vi "Main.vi"() -> ()   [LabVIEW 2010]
uses:
  vi.lib/Front Panel Layout/NI_SE_Front Panel Layout.lvlib
panel:
  in  "c":bool
  in  "b":bool
  in  "a":bool
  in  "Power":bool
  out "Sensor Data":dbl[](graph)
  in  "Config Keyword":string="small1"
  in  "cancel":bool
  in  "ok":bool
  # "The following values can be used for Config Keyword:\nsmall1\nsmall2\nlarge1"
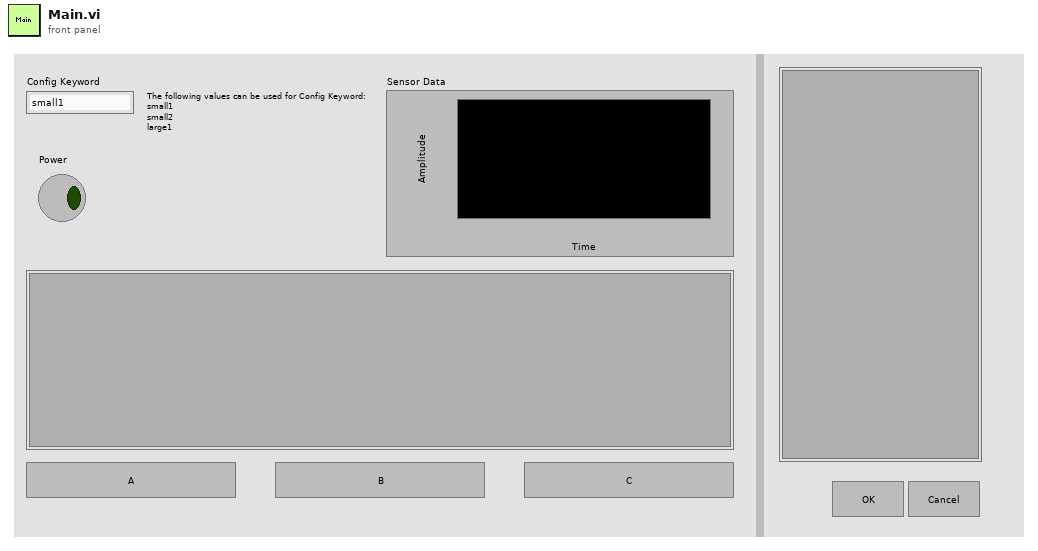
[diagram p1: front panel]
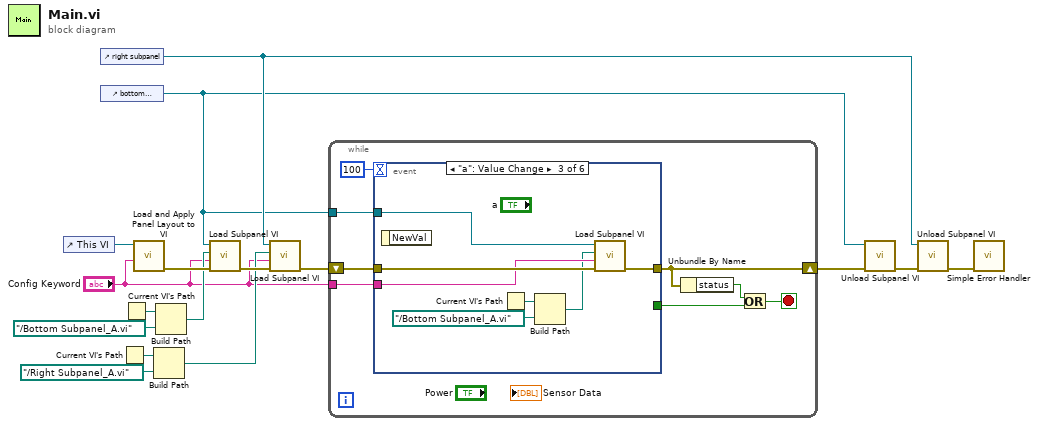
[diagram p0: block diagram]
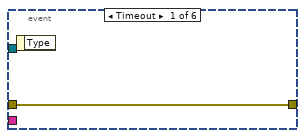
[diagram p2: hidden frame]
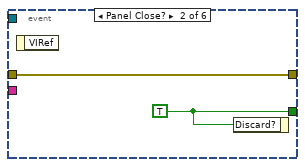
[diagram p3: hidden frame]
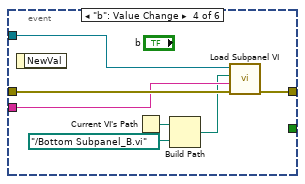
[diagram p4: hidden frame]
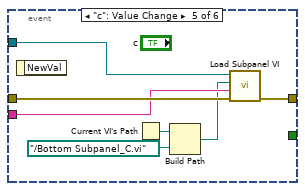
[diagram p5: hidden frame]
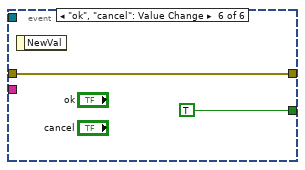
[diagram p6: hidden frame]
diagram:
  n1 = control-ref of="This VI"() -> (w16:refnum<vi>)
  n2 = control-ref of="right subpanel"() -> (w4:refnum<vi>)
  n3 = control-ref of="bottom subpanel"() -> (w3:refnum<vi>)
  n4 = Current VI's Path() -> (path=w7:path)
  n5 = Current VI's Path() -> (path=w15:path)
  n6 = call "Load and Apply Panel Layout to VI.vi"("keyword to match (\"\")"="Config Keyword", "VI refnum"=w16) -> ("error out"=w13:errorcluster)  [unwired: 8 in, 1 out]
  n7 = Build Path(base path=w7, name or relative path=path "../Right Subpanel_A.vi" ("path")) -> (appended path=w6:path)
  n8 = Build Path(base path=w15, name or relative path=path "../Bottom Subpanel_A.vi" ("path")) -> (appended path=w2:path)
  n9 = call "Load Subpanel VI.vi"("error in"=w13, "layout keyword"="Config Keyword", "subpanel VI path"=w2, "subpanel refnum"=w3) -> ("error out"=w9:errorcluster)  [unwired: 7 in]
  n10 = call "Load Subpanel VI.vi"("error in"=w9, "layout keyword"="Config Keyword", "subpanel VI path"=w6, "subpanel refnum"=w4) -> ("error out"=w8:errorcluster)  [unwired: 7 in]
  n11 = while {
    shift-right: [w22] -> w12
    shift-left: w8 -> [w24]
    tunnel: w3 -> [w19]
    tunnel: "Config Keyword" -> [w18]
    stop <- w21 stop-if-true
    n12 = event shown="[2] \"a\": Value Change" {
      selector: _ -> [_ _ _ _ _ _]
      dyn-events: _ -> [_ _ _ _ _ _]
      timeout: 100 -> [_ _ _ _ _ _]
      tunnel: w24 -> [w25 w27 w34 w41 w48 w50]
      tunnel: [w25 w27 w33 w40 w47 w50] -> w22
      tunnel: [_ w26 _ _ _ TRUE] -> w20
      tunnel: w19 -> [_ _ w31 w38 w45 _]
      tunnel: w18 -> [_ _ w32 w39 w46 _]
      event Timeout {
        n13 = event-data() -> ()  [unwired: 1 in, 1 out]
      }
      event Panel Close? {
        w26 = TRUE
        n14 = event-data() -> ()  [unwired: 1 in, 1 out]
        n15 = event-data("Discard?"=w26) -> ()  [unwired: 1 in, 1 out]
      }
      event "a": Value Change {
        n16 = event-data() -> ()  [unwired: 1 in, 1 out]
        n17 = Current VI's Path() -> (path=w30:path)
        n18 = Build Path(base path=w30, name or relative path=path "../Bottom Subpanel_A.vi" ("path")) -> (appended path=w29:path)
        n19 = call "Load Subpanel VI.vi"("error in"=w34, "layout keyword"=w32, "subpanel VI path"=w29, "subpanel refnum"=w31) -> ("error out"=w33:errorcluster)  [unwired: 7 in]
      }
      event "b": Value Change {
        n20 = event-data() -> ()  [unwired: 1 in, 1 out]
        n21 = Current VI's Path() -> (path=w37:path)
        n22 = Build Path(base path=w37, name or relative path=path "../Bottom Subpanel_B.vi" ("path")) -> (appended path=w36:path)
        n23 = call "Load Subpanel VI.vi"("error in"=w41, "layout keyword"=w39, "subpanel VI path"=w36, "subpanel refnum"=w38) -> ("error out"=w40:errorcluster)  [unwired: 7 in]
      }
      event "c": Value Change {
        n24 = event-data() -> ()  [unwired: 1 in, 1 out]
        n25 = Current VI's Path() -> (path=w44:path)
        n26 = Build Path(base path=w44, name or relative path=path "../Bottom Subpanel_C.vi" ("path")) -> (appended path=w43:path)
        n27 = call "Load Subpanel VI.vi"("error in"=w48, "layout keyword"=w46, "subpanel VI path"=w43, "subpanel refnum"=w45) -> ("error out"=w47:errorcluster)  [unwired: 7 in]
      }
      event "ok", "cancel": Value Change {
        n28 = event-data() -> ()  [unwired: 1 in, 1 out]
      }
    }
    n29 = Unbundle By Name(w22) -> ("status"=w17:bool)
    n30 = Or(x=w17, y=w20) -> (x .or. y?=w21:bool)
  }
  n31 = call "Unload Subpanel VI.vi"("error in"=w12, "subpanel refnum"=w3) -> ("error out"=w11:errorcluster)  [unwired: 9 in]
  n32 = call "Unload Subpanel VI.vi"("error in"=w11, "subpanel refnum"=w4) -> ("error out"=w10:errorcluster)  [unwired: 9 in]
  n33 = call <vilib>:"Simple Error Handler.vi"("error in (no error)"=w10) -> ()  [unwired: 4 in, 5 out]
